vi "GetSurfaceInfo.vi"(8 "No Error":errorcluster, 11 "Surface [SDL_Surface *]":i64) -> (0 "error out":errorcluster, 3 "Surface Info":T3 {"flag" items=["SDL_SURFACE_PREALLOCATED"=1, "SDL_SURFACE_LOCK_NEEDED"=2, "SDL_SURFACE_LOCKED"=4, "SDL_SURFACE_SIMD_ALIGNED"=8]})   [LabVIEW 2026, in "SDL3.lvlib" / "Surface.lvlib"]
doc: "<B>Summary</B>\nCreates a new surface identical to the existing surface.\n\n<B>Remarks</B>\nIf the original surface has alternate images, the new surface will have a reference to them as well.\n\nThe returned surface should be freed with SDL_DestroySurface()."
uses:
  Surface.lvlib
  SurfaceFlags--ring.ctl
  Pixels/PixelFormat--enum.ctl
  <vilib>/Utility/error.llb/Error Cluster From Error Code.vi
  LV-Utilities/LV-Utilities.lvlib
  Pixels/Pixels.lvlib
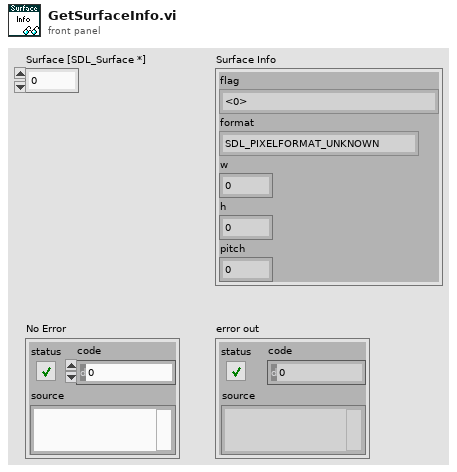
[diagram p1: front panel]
types:
  T1 = typedef "SDL3.lvlib/Surface.lvlib/SurfaceFlags--ring.ctl" = u32
  T2 = typedef "SDL3.lvlib/Pixels.lvlib/PixelFormat--enum.ctl" = enum32{"SDL_PIXELFORMAT_UNKNOWN", "SDL_PIXELFORMAT_INDEX1LSB", "SDL_PIXELFORMAT_INDEX1MSB", "SDL_PIXELFORMAT_INDEX2LSB", "SDL_PIXELFORMAT_INDEX2MSB", "SDL_PIXELFORMAT_INDEX4LSB", "SDL_PIXELFORMAT_INDEX4MSB", "SDL_PIXELFORMAT_INDEX8", "SDL_PIXELFORMAT_RGB332", "SDL_PIXELFORMAT_XRGB4444", "SDL_PIXELFORMAT_XBGR4444", "SDL_PIXELFORMAT_XRGB1555", "SDL_PIXELFORMAT_XBGR1555", "SDL_PIXELFORMAT_ARGB4444", "SDL_PIXELFORMAT_RGBA4444", "SDL_PIXELFORMAT_ABGR4444", "SDL_PIXELFORMAT_BGRA4444", "SDL_PIXELFORMAT_ARGB1555", "SDL_PIXELFORMAT_RGBA5551", "SDL_PIXELFORMAT_ABGR1555", "SDL_PIXELFORMAT_BGRA5551", "SDL_PIXELFORMAT_RGB565", "SDL_PIXELFORMAT_BGR565", "SDL_PIXELFORMAT_RGB24", "SDL_PIXELFORMAT_BGR24", "SDL_PIXELFORMAT_XRGB8888", "SDL_PIXELFORMAT_RGBX8888", "SDL_PIXELFORMAT_XBGR8888", "SDL_PIXELFORMAT_BGRX8888", "SDL_PIXELFORMAT_ARGB8888", "SDL_PIXELFORMAT_RGBA8888", "SDL_PIXELFORMAT_ABGR8888", "SDL_PIXELFORMAT_BGRA8888", "SDL_PIXELFORMAT_XRGB2101010", "SDL_PIXELFORMAT_XBGR2101010", "SDL_PIXELFORMAT_ARGB2101010", "SDL_PIXELFORMAT_ABGR2101010", "SDL_PIXELFORMAT_RGB48", "SDL_PIXELFORMAT_BGR48", "SDL_PIXELFORMAT_RGBA64", "SDL_PIXELFORMAT_ARGB64", "SDL_PIXELFORMAT_BGRA64", "SDL_PIXELFORMAT_ABGR64", "SDL_PIXELFORMAT_RGB48_FLOAT", "SDL_PIXELFORMAT_BGR48_FLOAT", "SDL_PIXELFORMAT_RGBA64_FLOAT", "SDL_PIXELFORMAT_ARGB64_FLOAT", "SDL_PIXELFORMAT_BGRA64_FLOAT", "SDL_PIXELFORMAT_ABGR64_FLOAT", "SDL_PIXELFORMAT_RGB96_FLOAT", "SDL_PIXELFORMAT_BGR96_FLOAT", "SDL_PIXELFORMAT_RGBA128_FLOAT", "SDL_PIXELFORMAT_ARGB128_FLOAT", "SDL_PIXELFORMAT_BGRA128_FLOAT", "SDL_PIXELFORMAT_ABGR128_FLOAT", "SDL_PIXELFORMAT_YV12", "SDL_PIXELFORMAT_IYUV", "SDL_PIXELFORMAT_YUY2", "SDL_PIXELFORMAT_UYVY", "SDL_PIXELFORMAT_YVYU", "SDL_PIXELFORMAT_NV12", "SDL_PIXELFORMAT_NV21", "SDL_PIXELFORMAT_P010", "SDL_PIXELFORMAT_EXTERNAL_OES"}
  T3 = cluster{"flag":T1, "format":T2, "w":i32, "h":i32, "pitch":i32}
  T4 = cluster{"Flag":T1, "Format":T2, "w":i32, "h":i32, "Pitch":i32}
  T5 = cluster{"flag":T1, "format":u32, "w":i32, "h":i32, "pitch":i32}
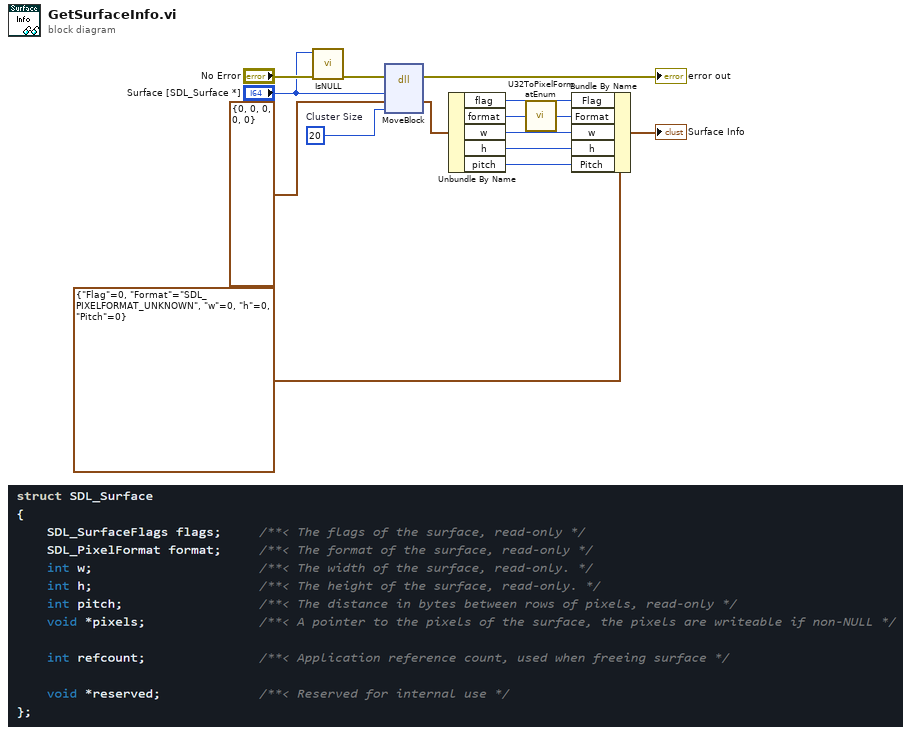
[diagram p0: block diagram]
diagram:
  w9 = 20  # Cluster Size
  n1 = call "IsNULL.vi"("error in (no error)"="No Error", "ptr"="Surface [SDL_Surface *]") -> ("error out"=w13:errorcluster)  [unwired: 9 in]
  n2 = dll-call lib="LabVIEW" fn="MoveBlock"(error in=w13, "Address"="Surface [SDL_Surface *]", "Destination"=T5 {"flag"=0, "format"=0, "w"=0, "h"=0, "pitch"=0}, "Size"=w9) -> (error out=→"error out":errorcluster, "Destination"=w8:T5)  [unwired: 5 in, 1 out]
  n3 = Unbundle By Name(w8) -> ("flag"=w6:T1, "format"=w4:u32, "w"=w5:i32, "h"=w2:i32, "pitch"=w1:i32)
  n4 = call "U32ToPixelFormatEnum.vi"("pixel_format_integer"=w4) -> ("pixel_format_enum"=w3:T2)
  n5 = Bundle By Name(cluster=T4 {"Flag"=0, "Format"=enum."SDL_PIXELFORMAT_UNKNOWN", "w"=0, "h"=0, "Pitch"=0}, "Flag"=w6, "Format"=w3, "w"=w5, "h"=w2, "Pitch"=w1) -> (→"Surface Info":T4)
